vi "ArrayToCluster.vi"(11 "Array":variant[](array[variant])) -> (3 "Cluster":variant)   [LabVIEW 2019]
doc: "JKI State Machine Objects (SMO) 1.3.0.56\nJKI - JKI\nCopyright (c) 2017, JKI"
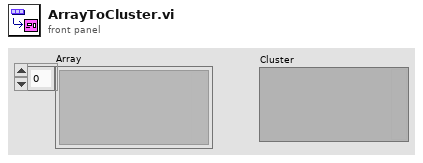
[diagram p1: front panel]
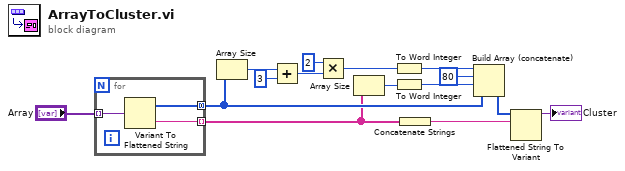
[diagram p0: block diagram]
diagram:
  n1 = for {
    tunnel: "Array" -> [w18] mode=indexing
    tunnel: [w17] -> w6 mode=concatenating
    tunnel: [w16] -> w4 mode=indexing
    n2 = Variant To Flattened String(Variant=w18) -> (data string=w16:string, 1:w17:i16[])
  }
  n3 = Array Size(array=w6) -> (size(s)=w2:i32)
  n4 = Add(x=w2, y=3) -> (x+y=w10:i32)
  n5 = Multiply(x=2, y=w10) -> (x*y=w8:i32)
  n6 = Array Size(array=w4) -> (size(s)=w3:i32)
  n7 = To Word Integer(number=w8) -> (16bit integer=w13:i16)
  n8 = To Word Integer(number=w3) -> (16bit integer=w12:i16)
  n9 = Concatenate Strings(w4) -> (w15:string)
  n10 = Build Array (concatenate)(w13, i16 80 ("number"), w12, w6) -> (w14:i16[])
  n11 = Flattened String To Variant(6:w15, 7:w14) -> (3:→"Cluster":variant)  [unwired: 1 in, 1 out]
